vi "2898 Updated drive.vi"() -> (0 "Aligning Mode?":bool, 2 "Shooter is Front":bool, 3 "Bridge Mode":bool)   [LabVIEW 2011]
uses:
  Team Code/Robot Global Data.vi
panel:
  in  "Turn Power":dbl=2.0
  in  "Align Divide":dbl=3.0
  in  "Deadzone":dbl=0.175
  in  "Drive Power":dbl=3.0
  in  "Bridge Divide":dbl=2.5
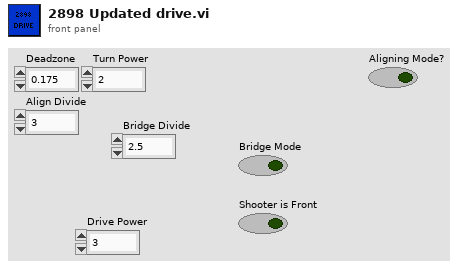
[diagram p1: front panel]
types:
  T1 = cluster{"Buttons":cluster{"A":bool, "B":bool, "X":bool, "Y":bool, "Left Bumper":bool, "Right Bumper":bool, "Back":bool, "Start":bool, "Left Thumbstick":bool, "Right Thumbstick":bool}, "Axes":cluster{"Left X ":dbl, "Left Y":dbl, "Triggers":dbl, "Right Stick X":dbl, "Right Stick Y":dbl, "D-Pad X":dbl}}
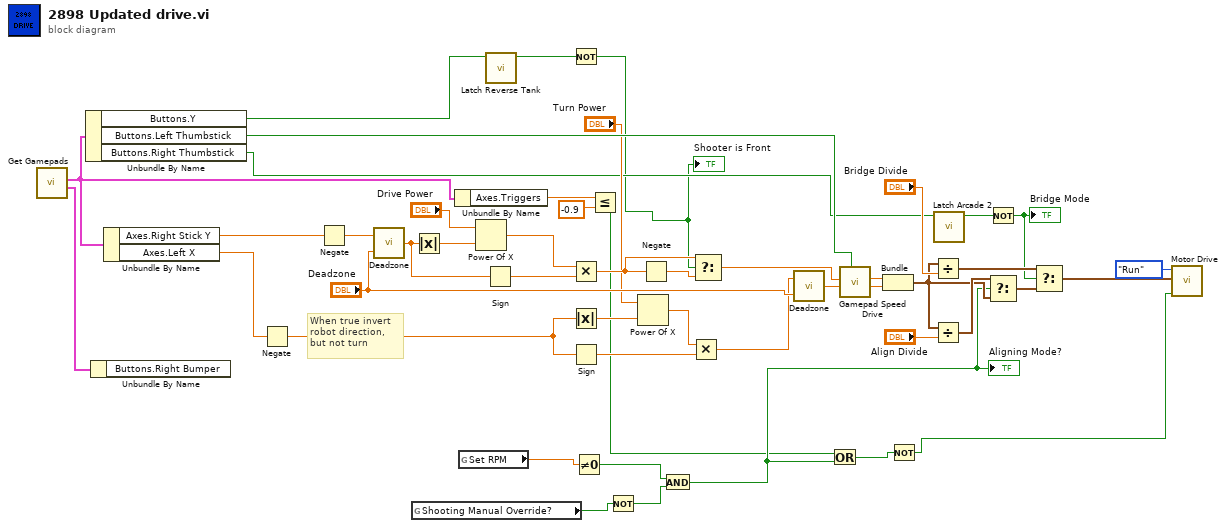
[diagram p0: block diagram]
diagram:
  # "When true invert robot direction, but not turn"
  n1 = call "Get Gamepads.vi"() -> ("Secondary"=w20:T1, "Driver"=w47:T1)  [unwired: 10 in]
  n2 = Unbundle By Name(w47) -> ("Buttons.Y"=w28:bool, "Buttons.Left Thumbstick"=w21:bool, "Buttons.Right Thumbstick"=w11:bool)
  n3 = Unbundle By Name(w20) -> ()  [unwired: 1 out]
  n4 = Unbundle By Name(w47) -> ("Axes.Right Stick Y"=w30:dbl, "Axes.Left X"=w29:dbl)
  n5 = Negate(x=w29) -> (-x=w15:dbl)
  n6 = Negate(x=w30) -> (-x=w46:dbl)
  n7 = call "Deadzone.vi"("Deadzone"="Deadzone", "Input"=w46) -> ("Output"=w43:dbl)
  n8 = global read "Robot Global Data.vi" "Shooting Manual Override?"() -> (w8:bool)
  n9 = Absolute Value(x=w43) -> (abs(x)=w40:dbl)
  n10 = Unbundle By Name(w47) -> ("Axes.Triggers"=w34:dbl)
  n11 = global read "Robot Global Data.vi" "Set RPM"() -> (w10:dbl)
  n12 = Power Of X(1:w40, 2:"Drive Power") -> (0:w39:dbl)
  n13 = Sign(1:w43) -> (0:w44:dbl)
  n14 = call "Latch Reverse Tank.vi"("Input"=w28) -> ("Latched"=w13:bool)  [unwired: 10 in]
  n15 = Not(x=w13) -> (.not. x?=w5:bool)
  "Shooter is Front" <- w5
  n16 = Multiply(x=w39, y=w44) -> (x*y=w45:dbl)
  n17 = Absolute Value(x=w15) -> (abs(x)=w18:dbl)
  n18 = Sign(1:w15) -> (0:w17:dbl)
  n19 = Not Equal To 0?(x=w10) -> (x != 0?=w9:bool)
  n20 = Less Or Equal?(x=w34, y=-0.9) -> (x <= y?=w3:bool)
  n21 = Not(x=w8) -> (.not. x?=w7:bool)
  n22 = Power Of X(1:w18, 2:"Turn Power") -> (0:w19:dbl)
  n23 = Negate(x=w45) -> (-x=w33:dbl)
  n24 = And(x=w9, y=w7) -> (x .and. y?=w4:bool)
  "Aligning Mode?" <- w4
  n25 = Multiply(x=w19, y=w17) -> (x*y=w14:dbl)
  n26 = Select(t=w45, s=w5, f=w33) -> (s? t:f=w32:dbl)
  n27 = call "Deadzone.vi"("Deadzone"="Deadzone", "Input"=w14) -> ("Output"=w31:dbl)
  n28 = Or(x=w3, y=w4) -> (x .or. y?=w2:bool)
  n29 = call "Gamepad Speed Drive.vi"("Quick Turn"=w21, "Turn"=w31, "Speed"=w32) -> ("Right Output"=w41:dbl, "Left Output"=w42:dbl)  [unwired: 7 out]
  n30 = Bundle("Left Output"=w42, "Right Output"=w41) -> (w23:cluster{"Left Output":dbl, "Right Output":dbl})  [unwired: 1 out]
  n31 = Not(x=w2) -> (.not. x?=w1:bool)
  n32 = Divide(x=w23, y="Bridge Divide") -> (x/y=w35:cluster{"Left Output":dbl, "Right Output":dbl})
  n33 = Divide(x=w23, y="Align Divide") -> (x/y=w24:cluster{"Left Output":dbl, "Right Output":dbl})
  n34 = call "Latch Arcade 2.vi"("Input"=w11) -> ("Latched"=w37:bool)  [unwired: 10 in]
  n35 = Not(x=w37) -> (.not. x?=w12:bool)
  "Bridge Mode" <- w12
  n36 = Select(t=w24, s=w4, f=w23) -> (s? t:f=w22:cluster{"Left Output":dbl, "Right Output":dbl})
  n37 = Select(t=w35, s=w12, f=w22) -> (s? t:f=w48:cluster{"Left Output":dbl, "Right Output":dbl})
  n38 = call "Motor Drive.vi"("Drive Around Mode?"=w1, "Motor Input"=w48, "Enum"=enum16{"Init", "Run", "SetBrakeCoast", "End"}."Run") -> ()  [unwired: 9 in]
